vi "Read Feed Forward.vi"(8 "Error In":errorcluster, 11 "Path":path) -> (0 "Error Out":errorcluster, 3 "Data Out":dbl[][](array[numeric]))   [LabVIEW 2013]
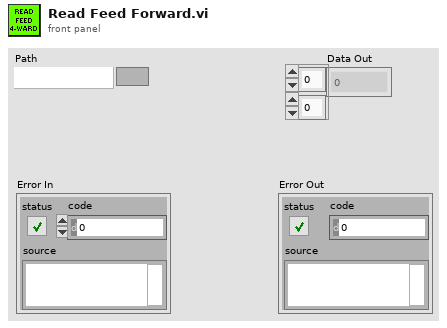
[diagram p1: front panel]
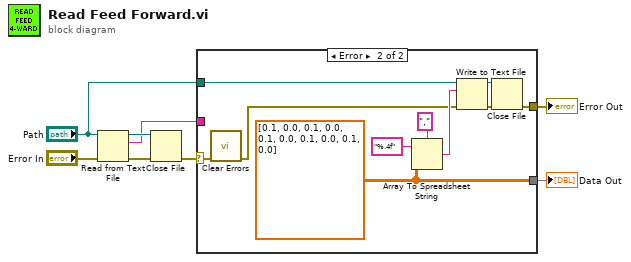
[diagram p0: block diagram]
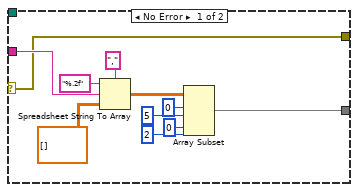
[diagram p2: hidden frame]
diagram:
  n1 = Read from Text File(file (use dialog)="Path", error in="Error In") -> (refnum out=w6:refnum<file>, text=w4:string, error out=w7:errorcluster)  [unwired: 2 in, 1 out]
  n2 = Close File(refnum=w6, error in=w7) -> (error out=w5:errorcluster)  [unwired: 1 out]
  n3 = case shown="Error" w5 {
    selector: w5 -> [w9 w29]
    tunnel: w4 -> [w17 _]
    tunnel: [w15 w26] -> w1
    tunnel: "Path" -> [_ w20]
    tunnel: [w9 w23] -> w2
    frame No Error {
      n4 = Spreadsheet String To Array(delimiter (Tab)=",", format string="%.2f", spreadsheet string=w17, array type (2D Dbl)=dbl[][] []) -> (array=w10:dbl[][])
      n5 = Array Subset(array=w10, index (row)=0 ("index"), length (row)=5 ("length"), index (col)=0 ("index"), length (col)=2 ("length")) -> (w15:dbl[][])
    }
    frame Error {
      w26 = dbl[][] [[0.1, 0.0], [0.1, 0.0], [0.1, 0.0], [0.1, 0.0], [0.1, 0.0]]
      n6 = call <vilib>:"Clear Errors.vi"("error in (no error)"=w29) -> ("error out"=w21:errorcluster)  [unwired: 6 in]
      n7 = Array To Spreadsheet String(delimiter (Tab)=",", array=w26, 3:"%.4f" ("format string")) -> (spreadsheet string=w25:string)
      n8 = Write to Text File(file (use dialog)=w20, text=w25, error in=w21) -> (refnum out=w28:refnum<file>, error out=w27:errorcluster)  [unwired: 1 in, 1 out]
      n9 = Close File(refnum=w28, error in=w27) -> (error out=w23:errorcluster)  [unwired: 1 out]
    }
  }
  "Error Out" <- w2
  "Data Out" <- w1
